vi "Get SMO Version.vi"(8 "error in (no error)":errorcluster, 11 "Instrument.Lockin in":refnum<class "Instrument.Lockin.lvclass">) -> (0 "error out":errorcluster, 2 "Version":string, 3 "Instrument.Lockin out":refnum<class "Instrument.Lockin.lvclass">)   [LabVIEW 2019, in "Instrument.Lockin.lvlib" / "Instrument.Lockin.lvclass"]
doc: "Override this VI to return the name of your Instrument"
uses:
  Instrument.Lockin.lvclass
  Lockin.Utilities/Lockin.Utilities.lvlib
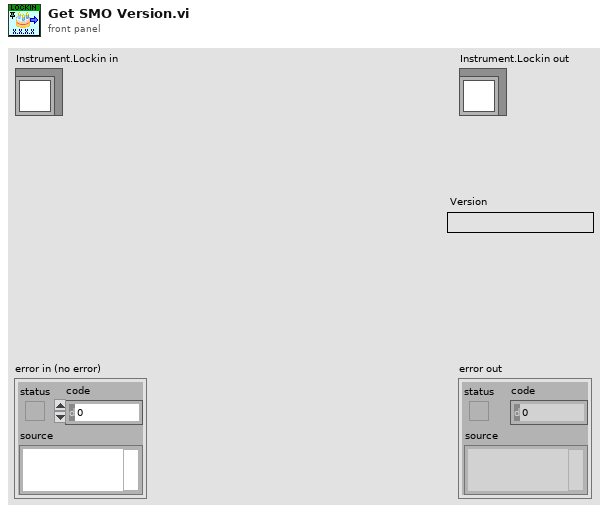
[diagram p1: front panel]
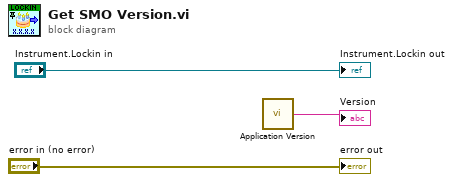
[diagram p0: block diagram]
diagram:
  n1 = call "Application Version.vi"() -> ("Version"=→"Version":string)
  "error out" <- "error in (no error)"
  "Instrument.Lockin out" <- "Instrument.Lockin in"
